vi "Test.vi"() -> ()   [LabVIEW 2009]
uses:
  <vilib>/vision/NI_Vision_Development_Module.lvlib
panel:
  in  "Size & Tolerance":T1={"X Size"=3, "Y Size"=3, "% Tolerance"=40}
  in  "stop 2":bool
  out "BlueEqLow":T2(plugin-control)
  out "BlueEq":T3(graph)
  out "BlueEq":T2(plugin-control)
  in  "stop":bool
  out "BlueEqLowThres":T2(plugin-control)
  out "Lum":T2(plugin-control)
  out "Sat":T2(plugin-control)
  out "Hue":T2(plugin-control)
  out "Blue":T2(plugin-control)
  out "Green":T2(plugin-control)
  out "Red":T2(plugin-control)
  in  "Manual":cluster{"Min":i32, "Max":i32}(slide)={"Min"=0, "Max"=150} caption="Threshold Range" scale=0.0..255.0
  out "Hue":T3(graph)
  out "Sat":T3(graph)
  out "Luma":T3(graph)
  out "Blue":T3(graph)
  out "Green":T3(graph)
  out "Red":T3(graph)
  out "Original":T2(plugin-control)
  in  "File Path":path
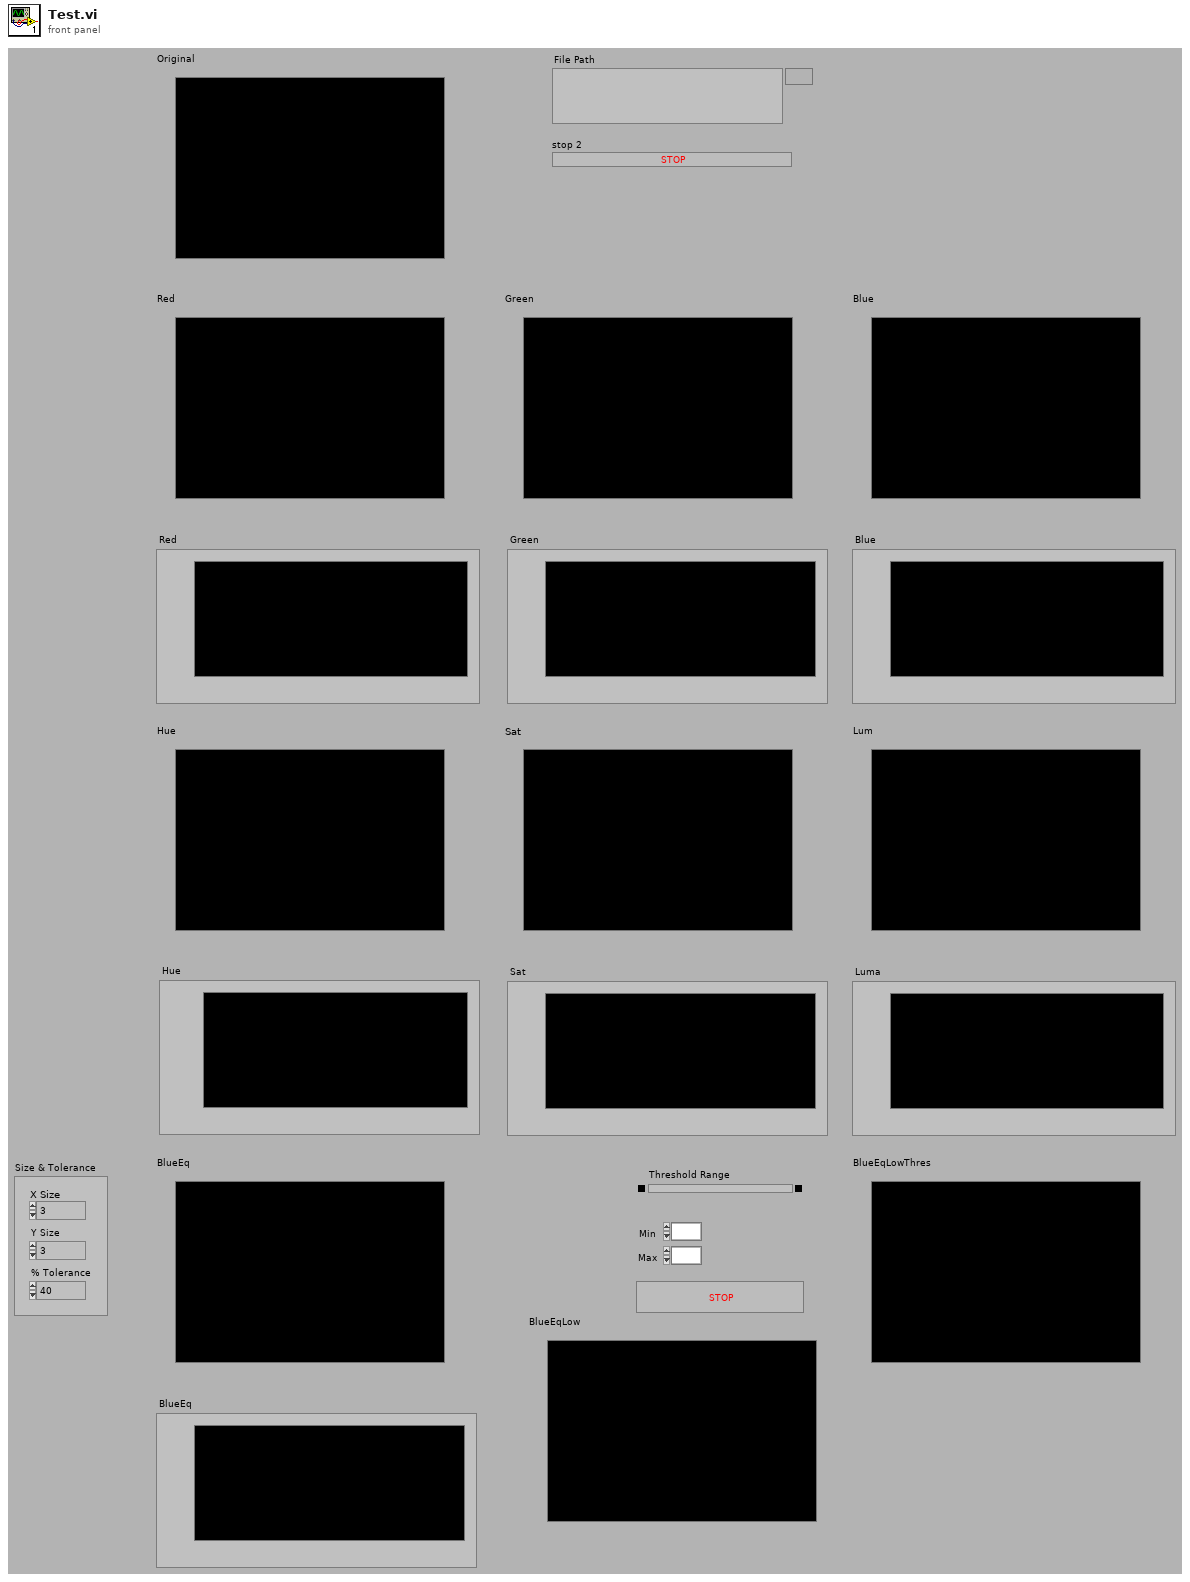
[diagram p1: front panel]
types:
  T1 = cluster{"X Size":i32, "Y Size":i32, "% Tolerance":i32}
  T2 = typedef "IMAQ Image.ctl" = refnum<image>
  T3 = cluster{"Starting Value":sgl, "Incremental Value":sgl, "Histogram":u32[]}
  T4 = typedef "Image Type" = u32
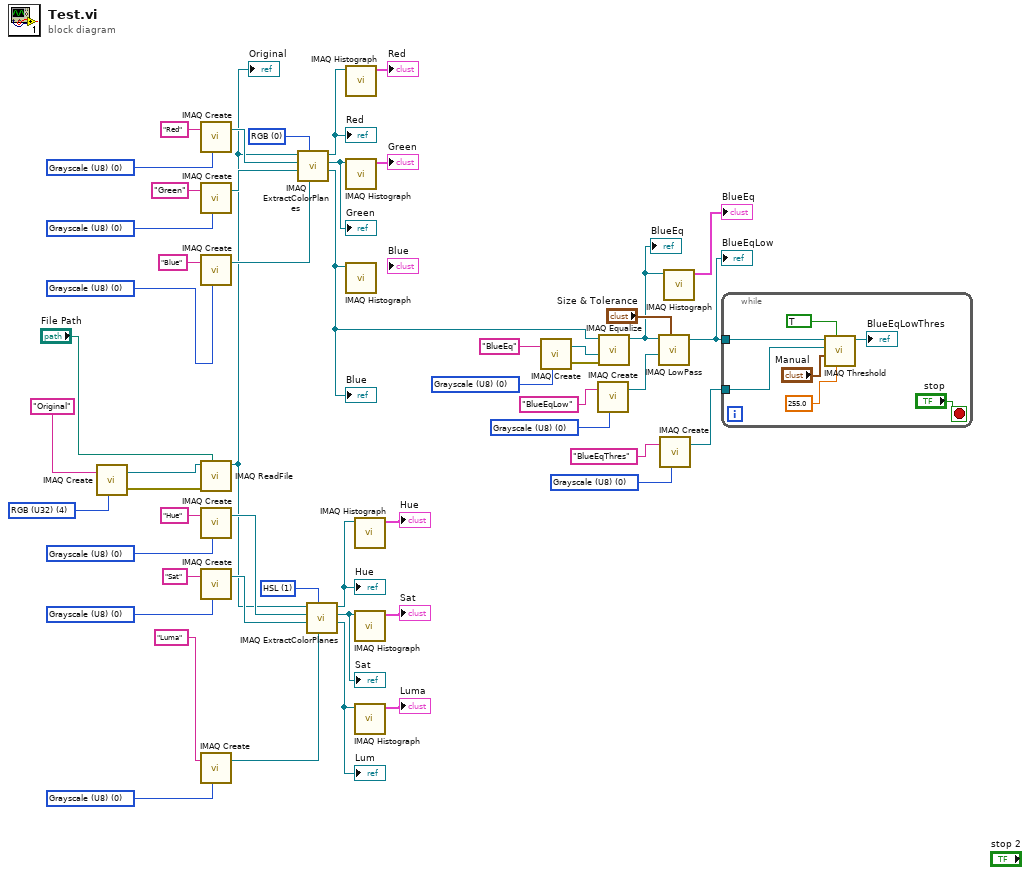
[diagram p0: block diagram]
diagram:
  w8 = T4 0 items=["Grayscale (U8)", "Grayscale (I16)", "Grayscale (SGL)", "Complex (CSG)", "RGB (U32)", "HSL (U32)", "RGB (U64)", "Grayscale (U16)"] ("Image Type")
  w12 = T4 0 items=["Grayscale (U8)", "Grayscale (I16)", "Grayscale (SGL)", "Complex (CSG)", "RGB (U32)", "HSL (U32)", "RGB (U64)", "Grayscale (U16)"] ("Image Type")
  w21 = T4 0 items=["Grayscale (U8)", "Grayscale (I16)", "Grayscale (SGL)", "Complex (CSG)", "RGB (U32)", "HSL (U32)", "RGB (U64)", "Grayscale (U16)"] ("Image Type")
  w37 = u16 1 items=["RGB", "HSL", "HSV", "HSI"] ("Color Mode")
  w32 = T4 0 items=["Grayscale (U8)", "Grayscale (I16)", "Grayscale (SGL)", "Complex (CSG)", "RGB (U32)", "HSL (U32)", "RGB (U64)", "Grayscale (U16)"] ("Image Type")
  w31 = T4 0 items=["Grayscale (U8)", "Grayscale (I16)", "Grayscale (SGL)", "Complex (CSG)", "RGB (U32)", "HSL (U32)", "RGB (U64)", "Grayscale (U16)"] ("Image Type")
  w28 = T4 0 items=["Grayscale (U8)", "Grayscale (I16)", "Grayscale (SGL)", "Complex (CSG)", "RGB (U32)", "HSL (U32)", "RGB (U64)", "Grayscale (U16)"] ("Image Type")
  w38 = u16 0 items=["RGB", "HSL", "HSV", "HSI"] ("Color Mode")
  w43 = T4 0 items=["Grayscale (U8)", "Grayscale (I16)", "Grayscale (SGL)", "Complex (CSG)", "RGB (U32)", "HSL (U32)", "RGB (U64)", "Grayscale (U16)"] ("Image Type")
  w44 = T4 0 items=["Grayscale (U8)", "Grayscale (I16)", "Grayscale (SGL)", "Complex (CSG)", "RGB (U32)", "HSL (U32)", "RGB (U64)", "Grayscale (U16)"] ("Image Type")
  w47 = T4 0 items=["Grayscale (U8)", "Grayscale (I16)", "Grayscale (SGL)", "Complex (CSG)", "RGB (U32)", "HSL (U32)", "RGB (U64)", "Grayscale (U16)"] ("Image Type")
  w48 = T4 4 items=["Grayscale (U8)", "Grayscale (I16)", "Grayscale (SGL)", "Complex (CSG)", "RGB (U32)", "HSL (U32)", "RGB (U64)", "Grayscale (U16)"] ("Image Type")
  n1 = call "IMAQ Create"("Image Name"="Original", "Image Type"=w48) -> ("New Image"=w50:T2, "error out"=w51:errorcluster)  [unwired: 3 in]
  n2 = call "IMAQ Create"("Image Name"="Red", "Image Type"=w47) -> ("New Image"=w41:T2)  [unwired: 3 in, 1 out]
  n3 = call "IMAQ Create"("Image Name"="Green", "Image Type"=w44) -> ("New Image"=w40:T2)  [unwired: 3 in, 1 out]
  n4 = call "IMAQ Create"("Image Name"="Blue", "Image Type"=w43) -> ("New Image"=w39:T2)  [unwired: 3 in, 1 out]
  n5 = call "IMAQ ReadFile"("File Path"="File Path", "error in (no error)"=w51, "Image"=w50) -> ("Image Out"=w27:T2)  [unwired: 4 in, 4 out]
  "Original" <- w27
  n6 = call "IMAQ Create"("Image Name"="Hue", "Image Type"=w28) -> ("New Image"=w34:T2)  [unwired: 3 in, 1 out]
  n7 = call "IMAQ Create"("Image Name"="Sat", "Image Type"=w31) -> ("New Image"=w35:T2)  [unwired: 3 in, 1 out]
  n8 = call "IMAQ Create"("Image Name"="Luma", "Image Type"=w32) -> ("New Image"=w36:T2)  [unwired: 3 in, 1 out]
  n9 = call "IMAQ ExtractColorPlanes"("Blue or Luma or Val or Inten Plane"=w39, "Color Mode"=w38, "Green or Sat Plane"=w40, "Red or Hue Plane"=w41, "Image Src"=w27) -> ("Blue or Luma or Val or Inten Plane out"=w3:T2, "Green or Sat Plane out"=w14:T2, "Red or Hue Plane out"=w17:T2)  [unwired: 3 in, 1 out]
  "Red" <- w17
  "Green" <- w14
  "Blue" <- w3
  n10 = call "IMAQ ExtractColorPlanes"("Blue or Luma or Val or Inten Plane"=w36, "Color Mode"=w37, "Green or Sat Plane"=w35, "Red or Hue Plane"=w34, "Image Src"=w27) -> ("Blue or Luma or Val or Inten Plane out"=w18:T2, "Green or Sat Plane out"=w16:T2, "Red or Hue Plane out"=w15:T2)  [unwired: 3 in, 1 out]
  "Hue" <- w15
  "Sat" <- w16
  "Lum" <- w18
  n11 = call "IMAQ Histograph"("Image"=w17) -> ("Histogram Graph"=→"Red":T3)  [unwired: 4 in, 6 out]
  n12 = call "IMAQ Histograph"("Image"=w14) -> ("Histogram Graph"=→"Green":T3)  [unwired: 4 in, 6 out]
  n13 = call "IMAQ Histograph"("Image"=w3) -> ()  [unwired: 4 in, 7 out]
  n14 = call "IMAQ Histograph"("Image"=w15) -> ("Histogram Graph"=→"Hue":T3)  [unwired: 4 in, 6 out]
  n15 = call "IMAQ Histograph"("Image"=w16) -> ("Histogram Graph"=→"Sat":T3)  [unwired: 4 in, 6 out]
  n16 = call "IMAQ Histograph"("Image"=w18) -> ("Histogram Graph"=→"Luma":T3)  [unwired: 4 in, 6 out]
  n17 = call "IMAQ Create"("Image Name"="BlueEq", "Image Type"=w12) -> ("New Image"=w11:T2, "error out"=w10:errorcluster)  [unwired: 3 in]
  n18 = call "IMAQ Create"("Image Name"="BlueEqLow", "Image Type"=w8) -> ("New Image"=w7:T2)  [unwired: 3 in, 1 out]
  n19 = call "IMAQ Equalize"("error in (no error)"=w10, "Image Dst"=w11, "Image Src"=w3) -> ("Image Dst Out"=w2:T2)  [unwired: 7 in, 1 out]
  "BlueEq" <- w2
  n20 = call "IMAQ LowPass"("Image Src"=w2, "Size & Tolerance"="Size & Tolerance", "Image Dst"=w7) -> ("Image Dst Out"=w1:T2)  [unwired: 4 in, 1 out]
  "BlueEqLow" <- w1
  n21 = call "IMAQ Create"("Image Name"="BlueEqThres", "Image Type"=w21) -> ("New Image"=w19:T2)  [unwired: 3 in, 1 out]
  n22 = call "IMAQ Histograph"("Image"=w2) -> ("Histogram Graph"=→"BlueEq":T3)  [unwired: 4 in, 6 out]
  n23 = while {
    tunnel: w19 -> [w58]
    tunnel: w1 -> [w57]
    stop <- "stop" stop-if-true
    n24 = call "IMAQ Threshold"("Replace Value"=sgl 255.0, "Keep/Replace Value (Replace)"=TRUE, "Range"="Manual", "Image Dst"=w58, "Image Src"=w57) -> ("Image Dst Out"=→"BlueEqLowThres":T2)  [unwired: 5 in, 1 out]
  }
